vi "DialogAddDesignPattern.vi"(0 "ClassWriterNative":refnum<class "ClassWriterNative.lvclass">, 1 "ClassItemRefIn":refnum<vi>, 5 "error in (no error)":errorcluster) -> (14 "ClassWriterNative":refnum<class "ClassWriterNative.lvclass">, 15 "ClassItemRefOut":refnum<vi>, 16 "AddDesignPatternData":T2, 17 "Cancelled":bool, 19 "error out":errorcluster)   [LabVIEW 2014, in "ClassWriterNative.lvclass"]
uses:
  <resource>/Framework/Providers/Open_GDS/ClassProviders/Provider_LvNativeClass/ClassWriterNative_class/ClassWriterNative.lvclass
  <resource>/Framework/Providers/Open_GDS/ClassProviders/Provider_BaseClassInterface/AddDesignPatternData.ctl
  <resource>/Framework/Providers/Open_GDS/SubVIs/GOOP_HelpButton.ctl
  <resource>/Framework/Providers/Open_GDS/ClassProviders/Provider_BaseClassInterface/DesignPatternsData.ctl
  <resource>/Framework/Providers/Open_GDS/ClassProviders/Common/LvClass_class/GDSLvClass_PlugIn.ctl
  <resource>/Framework/Providers/Open_GDS/ClassProviders/Common/LvClass_class/GDSLvClass_PlugInTypes.ctl
  <resource>/Framework/Providers/Open_GDS/ClassProviders/Provider_BaseClassInterface/BaseProvider_SubVIs/BaseProvider_DesignPatternsActions.ctl
panel:
  out "ProductPicture":picture
  out "TextError":string
  out "_Description":string caption="Description"
  in  "_DesignPatterns":string(tree) caption="Design Patterns"
  out "_ClassTemplateUsed":string caption="Class Template Used"
  out "_ClassProviderName":string caption="Class Provider Name"
  out "_ClassName":string caption="Class name"
  in  "_HelpCreateMethod":T1
  in  "_Help":bool
  in  "_Cancel":bool
  in  "_Next>>":bool
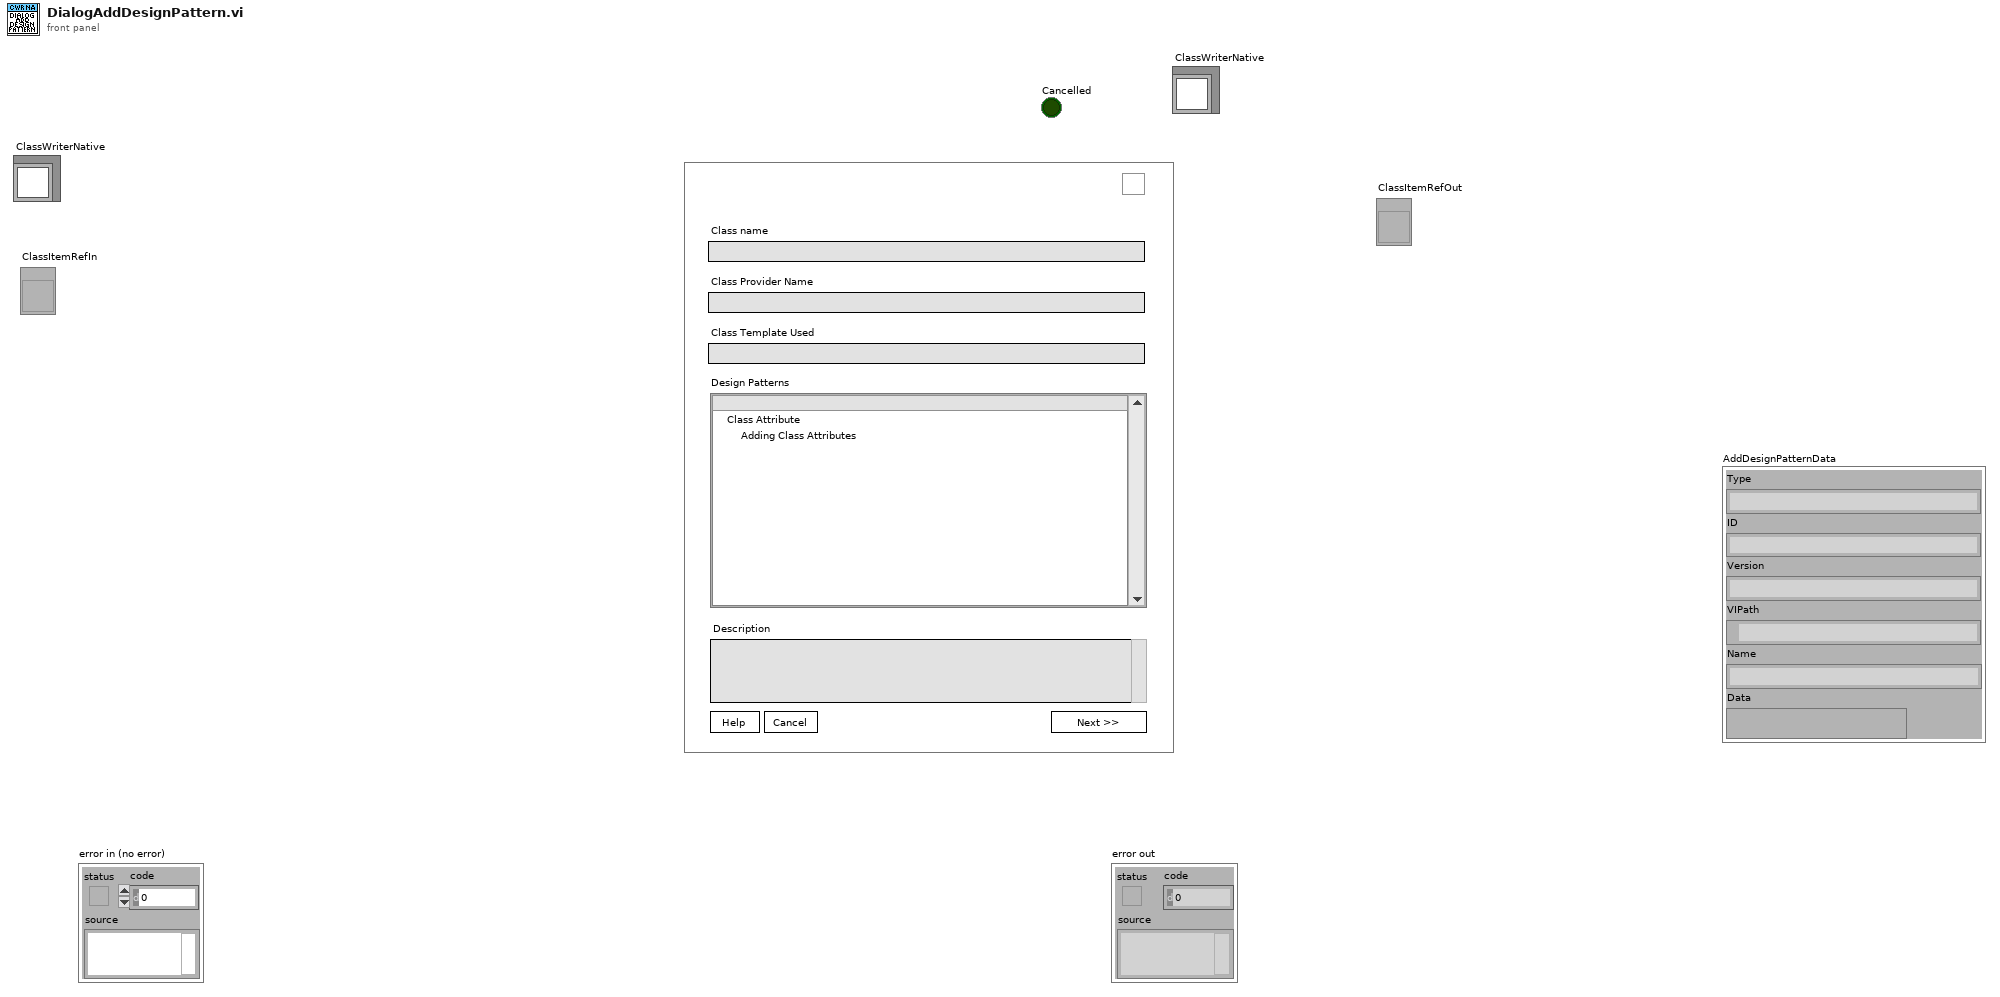
[diagram p1: front panel]
types:
  T1 = typedef "GOOP_HelpButton.ctl" = bool
  T2 = typedef "AddDesignPatternData.ctl" = cluster{"Type":string, "ID":string, "Version":string, "VIPath":path, "Name":string, "Data":variant}
  T3 = typedef "DesignPatternsData.ctl" = cluster{"Type":string, "Patterns":cluster{"ID":string, "Path":path, "Name":string, "Desc":string, "Version":string, "DependenciesID":string[], "OnlyOne":bool}[]}
  T4 = cluster{"Cancel":bool, "ClassProviderName":string, "ClassTemplateUsed":string, "DesignPatterns":T3[], "DataOut":variant, "PlugInVI":path, "DesignPatternID":string, "DesignPatternType":string, "PlugInIDs":string[], "DesignPatternVer":string, "Name":string}
  T5 = typedef "BaseProvider_DesignPatternsActions.ctl" = enum16{"AddPatternDialog", "GeneratePattern", "RemovePattern", "CreatePatternMethod", "UpdatePattern"}
  T6 = typedef "GDSLvClass_PlugIn.ctl" = cluster{"Type":T7, "ID":string, "Version":string, "Path":path, "Name":string, "Data":variant}
  T7 = typedef "GDSLvClass_PlugInTypes.ctl" = enum16{"DesignPattern", "MethodTypes"}
  T8 = typedef "GDSLvCLass_ClassSettingsType.ctl" = cluster{"ClassProviderName":string, "ClassTemplateUsed":string, "ClassTemplateVersion":string, "ClassDescription":string, "PlugIns":T6[], "ConnectorPanePattern":string}
  T9 = cluster{"ID":string, "Path":path, "Name":string, "Desc":string, "Version":string, "DependenciesID":string[], "OnlyOne":bool}[]
  T10 = cluster{"ID":string, "Path":path, "Name":string, "Desc":string, "Version":string, "DependenciesID":string[], "OnlyOne":bool}
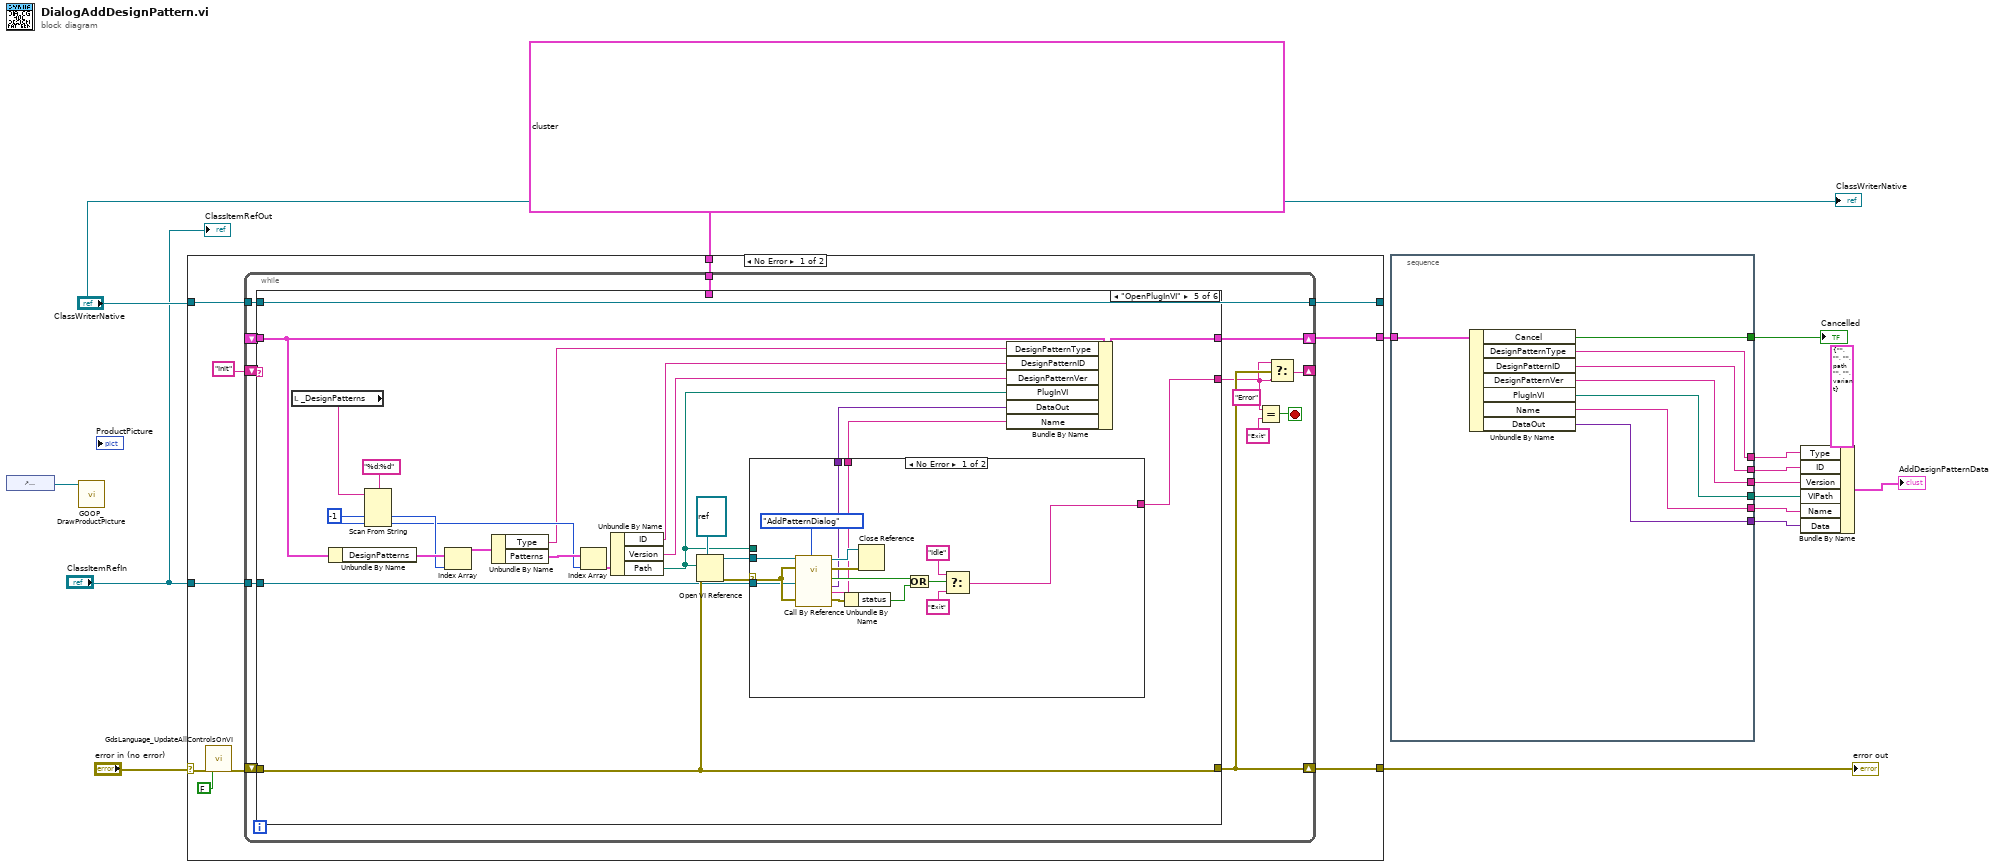
[diagram p0: block diagram]
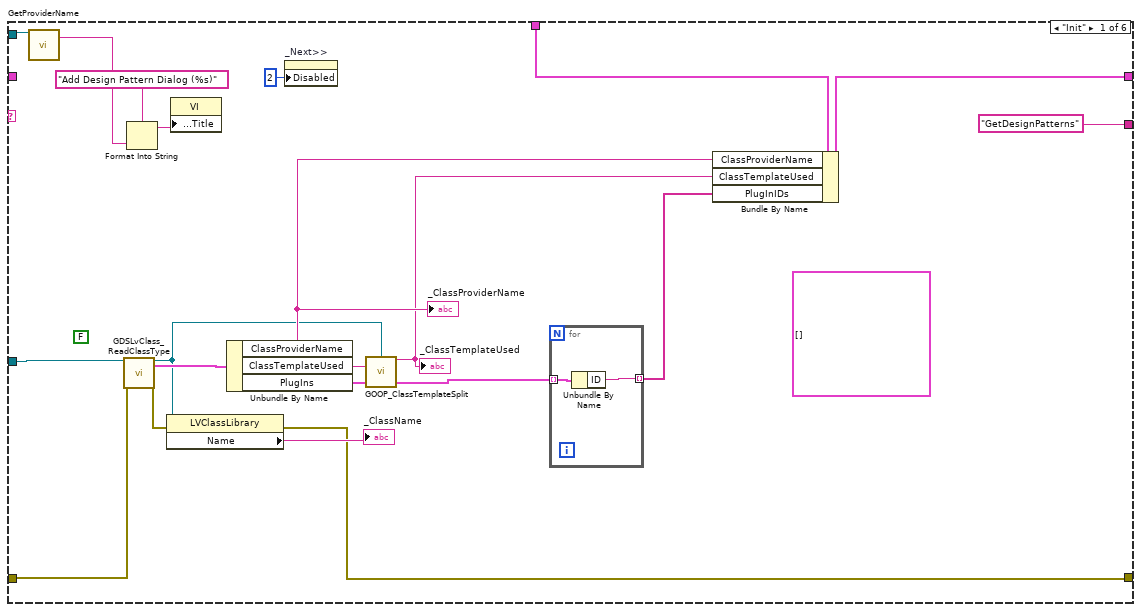
[diagram p2: hidden frame]
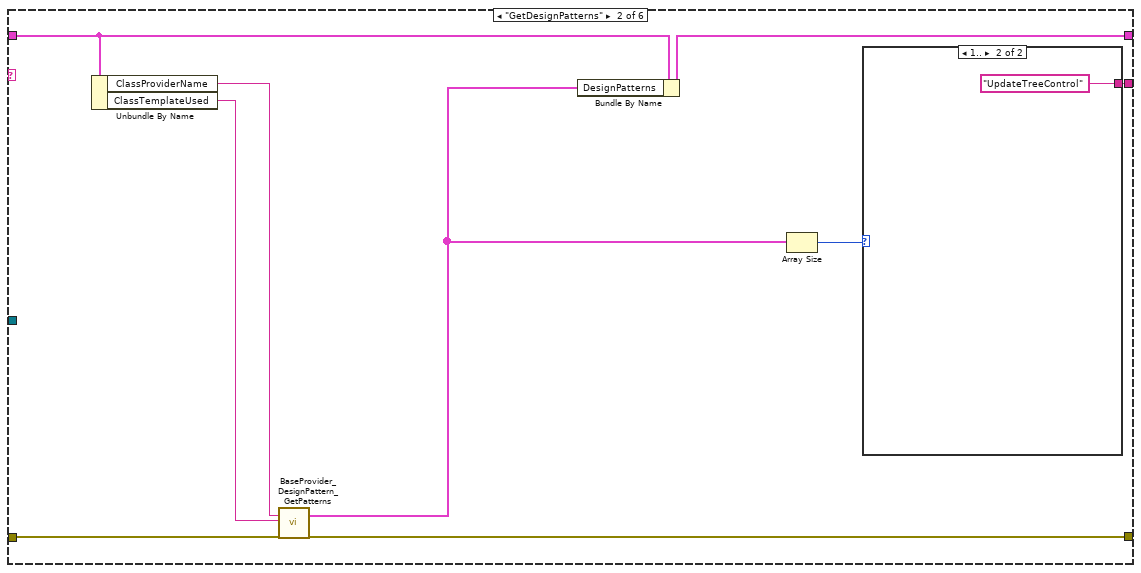
[diagram p3: hidden frame]
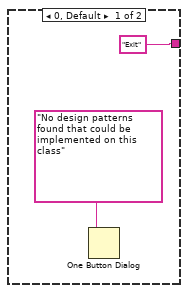
[diagram p4: hidden frame]
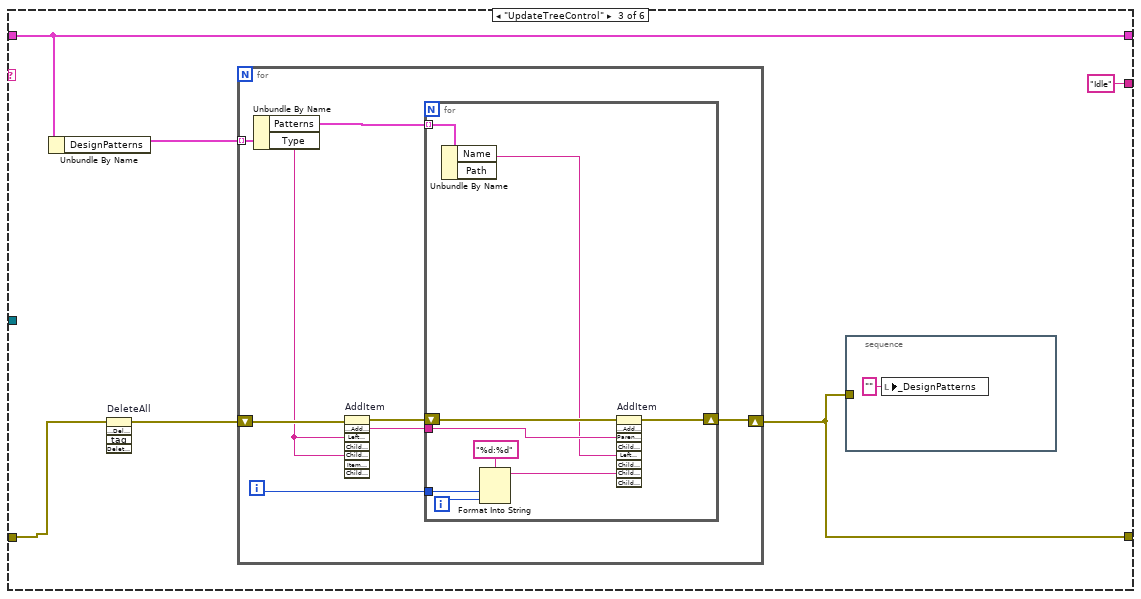
[diagram p5: hidden frame]
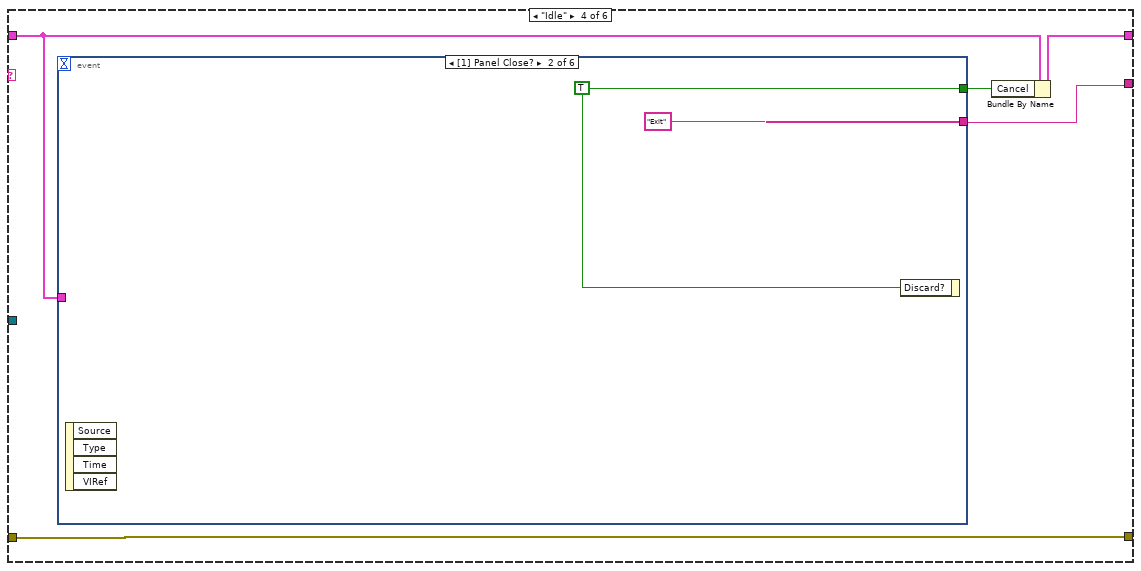
[diagram p6: hidden frame]
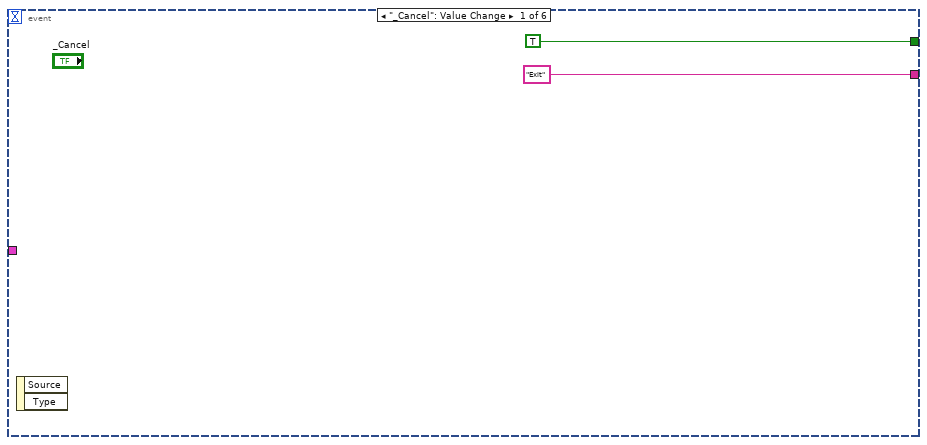
[diagram p7: hidden frame]
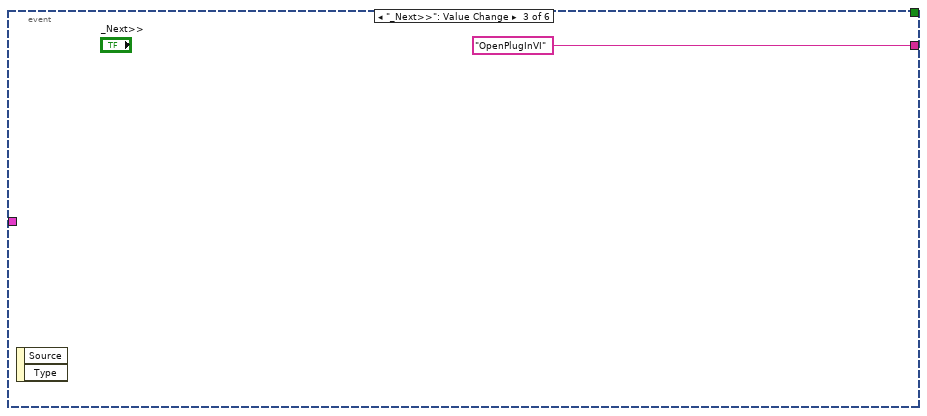
[diagram p8: hidden frame]
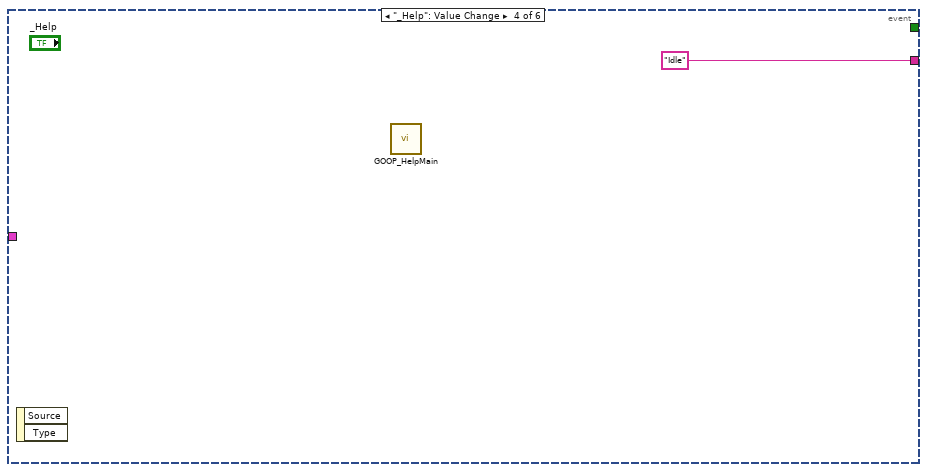
[diagram p9: hidden frame]
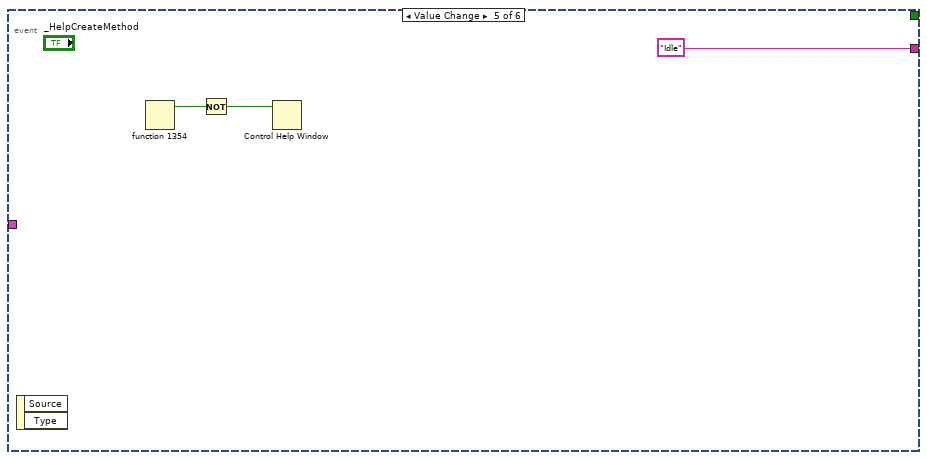
[diagram p10: hidden frame]
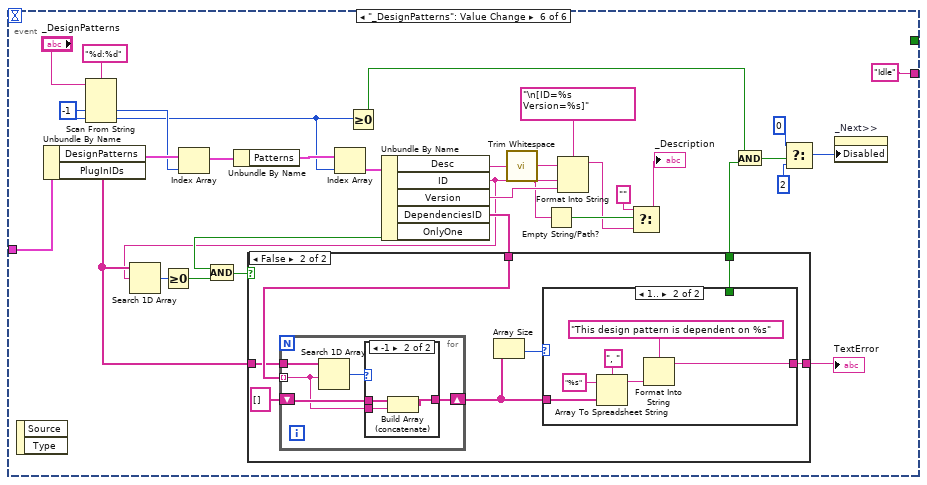
[diagram p11: hidden frame]
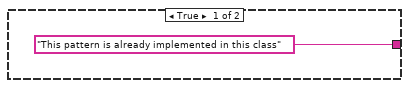
[diagram p12: hidden frame]
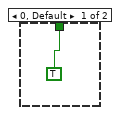
[diagram p13: hidden frame]
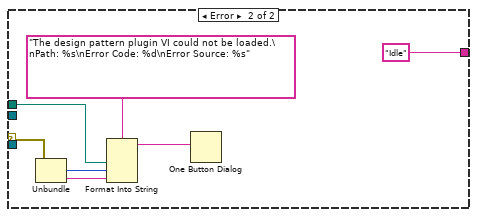
[diagram p15: hidden frame]
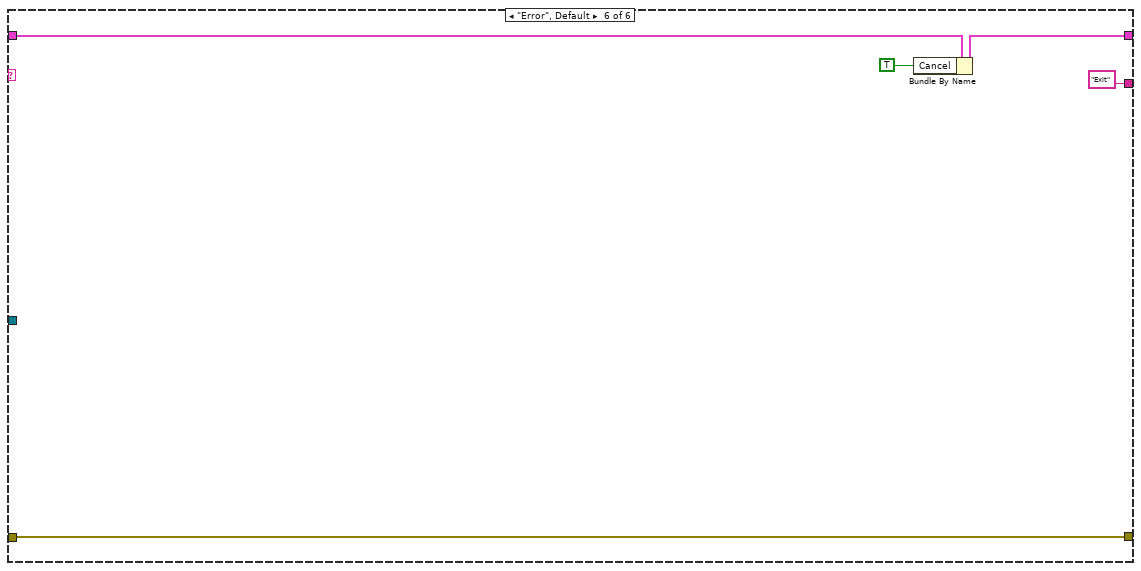
[diagram p16: hidden frame]
diagram:
  n1 = control-ref of="ProductPicture"() -> (w1:refnum<vi>)
  n2 = call <resource>:"GOOP_DrawProductPicture.vi"("ProductPictureControl"=w1) -> ()  [unwired: 10 in, 1 out]
  n3 = case shown="No Error" "error in (no error)" {
    selector: "error in (no error)" -> [w19 w220]
    tunnel: "ClassWriterNative" -> [w23 w219]
    tunnel: [w26 w220] -> w13
    tunnel: [w24 w219] -> _
    tunnel: T4 {"Cancel"=FALSE, "ClassProviderName"="", "ClassTemplateUsed"="", "DesignPatterns"=[], "DataOut"=variant, "PlugInVI"=path "", "DesignPatternID"="", "DesignPatternType"="", "PlugInIDs"=[], "DesignPatternVer"="", "Name"=""} ("output cluster") -> [w22 _]
    tunnel: "ClassItemRefIn" -> [w21 _]
    tunnel: [w20 _] -> w15
    frame No Error {
      n4 = call <resource>:"GdsLanguage_UpdateAllControlsOnVI.vi"("error in (no error)"=w19, "CreateLanguageFile(Use this to create a languageFile)"=FALSE) -> ("error out"=w18:errorcluster)  [unwired: 16 in, 1 out]
      n5 = while {
        shift-right: [w33] -> w26
        shift-left: w18 -> [w39]
        shift-right: [w32] -> _
        shift-left: "Init" -> [w36]
        shift-right: [w37] -> w20
        shift-left: _ -> [w38]
        tunnel: w23 -> [w29]
        tunnel: [w29] -> w24
        tunnel: w22 -> [w28]
        tunnel: w21 -> [w27]
        stop <- w34 stop-if-true
        n6 = case shown="\"OpenPlugInVI\"" w36 {
          tunnel: w38 -> [_ w63 w78 w98 w181 w216]
          tunnel: [w45 w62 w78 w100 w179 w215] -> w37
          tunnel: w39 -> [w52 w68 w77 w102 w178 w217]
          tunnel: [w48 w65 w74 w102 w178 w217] -> w33
          tunnel: w29 -> [w55 _ _ _ _ _]
          tunnel: ["GetDesignPatterns" w70 "Idle" w101 w176 "Exit"] -> w31
          tunnel: w28 -> [w46 _ _ _ _ _]
          tunnel: w27 -> [w53 _ _ _ w173 _]
          frame "Init" {
            (unwired) T6[] [] ("PlugIns")
            (unwired) FALSE ("Visible")
            n7 = call-dynamic "GetProviderName.vi"("ClassWriterNative in"=w55) -> ("ProviderName"=w54:string)  [unwired: 16 in, 2 out]
            n8 = call <resource>:"GDSLvClass_ReadClassType.vi"("Class Refnum In"=w53, "error in (no error)"=w52) -> ("Class Refnum Out"=w40:refnum<vi>, "ClassSettings"=w51:T8, "error out"=w49:errorcluster)  [unwired: 15 in]
            n9 = Format Into String(format string="Add Design Pattern Dialog (%s)", w54) -> (resulting string=w57:string)  [unwired: 2 in, 1 out]
            n10 = property class="LVClassLibrary"(reference=w40, error in=w49) -> (error out=w48:errorcluster, "Name"=→"_ClassName":string)  [unwired: 1 out]
            n11 = property class="VI"("Front Panel.Title"=w57) -> ()  [unwired: 2 in, 2 out]
            n12 = Unbundle By Name(w51) -> ("ClassProviderName"=w47:string, "ClassTemplateUsed"=w42:string, "PlugIns"=w44:T6[])
            "_ClassProviderName" <- w47
            n13 = property on="_Next>>" class="Bool"("Disabled"=u8 2) -> ()  [unwired: 2 in, 2 out]
            n14 = call <resource>:"GOOP_ClassTemplateSplit.vi"("ClassItemRefIn"=w40, "FullClassTemplate"=w42) -> ("StandardTemplate"=w41:string)  [unwired: 12 in, 1 out]
            "_ClassTemplateUsed" <- w41
            n15 = for {
              tunnel: w44 -> [w61] mode=indexing
              tunnel: [w60] -> w43 mode=indexing
              n16 = Unbundle By Name(w61) -> ("ID"=w60:string)
            }
            n17 = Bundle By Name(cluster=w46, "ClassProviderName"=w47, "ClassTemplateUsed"=w41, "PlugInIDs"=w43) -> (w45:T4)
          }
          frame "GetDesignPatterns" {
            n18 = Unbundle By Name(w63) -> ("ClassProviderName"=w67:string, "ClassTemplateUsed"=w66:string)
            n19 = call <resource>:"BaseProvider_DesignPattern_GetPatterns.vi"("FilterOnProviders(Ignored If Empty)"=w67, "FilterOnTemplate(Ignored If Empty)"=w66, "error in (no error)"=w68) -> ("DesignPatterns"=w64:T3[], "error out"=w65:errorcluster)  [unwired: 15 in]
            n20 = Bundle By Name(cluster=w63, "DesignPatterns"=w64) -> (w62:T4)
            n21 = Array Size(array=w64) -> (size(s)=w69:i32)
            n22 = case shown="1.." w69 {
              tunnel: ["Exit" "UpdateTreeControl"] -> w70
              frame 0, Default {
                n23 = One Button Dialog(message="No design patterns found that could be implemented on this class" ("format string")) -> ()  [unwired: 1 in, 1 out]
              }
              frame 1.. {
              }
            }
          }
          frame "UpdateTreeControl" {
            n24 = Unbundle By Name(w78) -> ("DesignPatterns"=w75:T3[])
            n25 = invoke on="DeleteAll" class="Tree (strict)" method="Edit Tree Items.Delete"(error in=w77) -> (error out=w76:errorcluster)  [unwired: 4 in, 4 out]
            n26 = for {
              shift-right: [w81] -> w74
              shift-left: w76 -> [w88]
              tunnel: w75 -> [w87] mode=indexing
              i -> [w82]
              n27 = Unbundle By Name(w87) -> ("Patterns"=w83:T9, "Type"=w84:string)
              n28 = invoke on="AddItem" class="Tree (strict)" method="Edit Tree Items.Add Item to End"(error in=w88, "Left Cell"=w84, "Child Tag"=w84) -> (error out=w86:errorcluster, "Edit Tree Items:Add Item to End"=w85:string)  [unwired: 5 in, 6 out]
              n29 = for {
                shift-right: [w89] -> w81
                shift-left: w86 -> [w96]
                tunnel: w85 -> [w97]
                tunnel: w83 -> [w95] mode=indexing
                tunnel: w82 -> [w92]
                i -> [w91]
                n30 = Unbundle By Name(w95) -> ("Name"=w94:string)  [unwired: 1 out]
                n31 = Format Into String(format string="%d:%d", w92, w91) -> (resulting string=w90:string)  [unwired: 2 in, 1 out]
                n32 = invoke on="AddItem" class="Tree (strict)" method="Edit Tree Items.Add Item"(error in=w96, "Parent Tag"=w97, "Left Cell"=w94, "Child Tag"=w90) -> (error out=w89:errorcluster)  [unwired: 5 in, 8 out]
              }
            }
            n33 = stacked-sequence {
              tunnel: w74 -> [_]
              frame #0 {
                n34 = local write "_DesignPatterns"("" ("_DesignPatterns")) -> ()
              }
            }
          }
          frame "Idle" {
            n35 = event shown="[1] Panel Close?" {
              selector: _ -> [_ _ _ _ _ _]
              dyn-events: _ -> [_ _ _ _ _ _]
              timeout: _ -> [_ _ _ _ _ _]
              tunnel: ["Exit" "Exit" "OpenPlugInVI" "Idle" "Idle" "Idle"] -> w101
              tunnel: [TRUE w105 _ _ _ _] -> w99
              tunnel: w98 -> [_ _ _ _ _ w143]
              event "_Cancel": Value Change {
                n36 = event-data() -> ()  [unwired: 1 in, 2 out]
              }
              event Panel Close? {
                w105 = TRUE
                n37 = event-data() -> ()  [unwired: 1 in, 4 out]
                n38 = event-data("Discard?"=w105) -> ()  [unwired: 1 in, 1 out]
              }
              event "_Next>>": Value Change {
                n39 = event-data() -> ()  [unwired: 1 in, 2 out]
              }
              event "_Help": Value Change {
                n40 = event-data() -> ()  [unwired: 1 in, 2 out]
                n41 = call <resource>:"GOOP_HelpMain.vi"() -> ()  [unwired: 12 in]
              }
              event Value Change {
                n42 = event-data() -> ()  [unwired: 1 in, 2 out]
                n43 = fn#1354() -> (1:w111:bool)  [unwired: 1 out]
                n44 = Not(x=w111) -> (.not. x?=w110:bool)
                n45 = Control Help Window(1:w110) -> ()  [unwired: 1 in]
              }
              event "_DesignPatterns": Value Change {
                w131 = -1 ("default value 1")
                n46 = event-data() -> ()  [unwired: 1 in, 2 out]
                n47 = Unbundle By Name(w143) -> ("DesignPatterns"=w142:T3[], "PlugInIDs"=w121:string[])
                n48 = Scan From String(format string="%d:%d", input string="_DesignPatterns", default 1=w131, default 2=w131) -> (output 1=w141:i32, output 2=w138:i32)  [unwired: 2 in, 3 out]
                n49 = Index Array(array=w142, index=w141) -> (element=w140:T3)
                n50 = Unbundle By Name(w140) -> ("Patterns"=w139:T9)
                n51 = Index Array(array=w139, index=w138) -> (element=w136:T10)
                n52 = Greater Or Equal To 0?(x=w138) -> (x >= 0?=w126:bool)
                n53 = Unbundle By Name(w136) -> ("Desc"=w130:string, "ID"=w115:string, "Version"=w123:string, "DependenciesID"=w128:string[], "OnlyOne"=w117:bool)
                n54 = Search 1D Array(1D array=w121, element=w115) -> (index of element=w120:i32)  [unwired: 1 in]
                n55 = Greater Or Equal To 0?(x=w120) -> (x >= 0?=w119:bool)
                n56 = Compound Arithmetic op=AND(w117, w119) -> (w118:bool)
                n57 = case shown="False" w118 {
                  tunnel: w128 -> [_ w152]
                  tunnel: ["This pattern is already implemented in this class" w149] -> w127
                  tunnel: [_ w147] -> w124
                  tunnel: w121 -> [_ w146]
                  frame True {
                  }
                  frame False {
                    n58 = for {
                      tunnel: w152 -> [w161] mode=indexing
                      tunnel: w146 -> [w164]
                      shift-right: [w160] -> w150
                      shift-left: string[] [] -> [w162]
                      n59 = Search 1D Array(1D array=w164, element=w161) -> (index of element=w163:i32)  [unwired: 1 in]
                      n60 = case shown="-1" w163 {
                        tunnel: w162 -> [w165 w168]
                        tunnel: w161 -> [_ w167]
                        tunnel: [w165 w166] -> w160
                        frame Default {
                        }
                        frame -1 {
                          n61 = Build Array (concatenate)(w168, w167) -> (w166:string[])
                        }
                      }
                    }
                    n62 = Array Size(array=w150) -> (size(s)=w148:i32)
                    n63 = case shown="1.." w148 {
                      tunnel: w150 -> [_ w159]
                      tunnel: [_ w154] -> w149
                      tunnel: [TRUE _] -> w147
                      frame 0, Default {
                      }
                      frame 1.. {
                        n64 = Array To Spreadsheet String(delimiter (Tab)=", ", array=w159, 3:"%s" ("format string")) -> (spreadsheet string=w156:string)
                        n65 = Format Into String(format string="This design pattern is dependent on %s", w156) -> (resulting string=w154:string)  [unwired: 2 in, 1 out]
                      }
                    }
                  }
                }
                "TextError" <- w127
                n66 = call <vilib>:"Trim Whitespace.vi"("string"=w130) -> ("trimmed string"=w129:string)  [unwired: 1 in]
                n67 = Empty String/Path?(string/path=w115) -> (empty?=w116:bool)
                n68 = Format Into String(format string="\n[ID=%s Version=%s]", initial string=w129, w115, w123) -> (resulting string=w114:string)  [unwired: 1 in, 1 out]
                n69 = Select(t="" ("ID"), s=w116, f=w114) -> (s? t:f=→"_Description":string)
                n70 = And(x=w126, y=w124) -> (x .and. y?=w125:bool)
                n71 = Select(t=u8 0, s=w125, f=u8 2 ("Disabled")) -> (s? t:f=w133:u8)
                n72 = property on="_Next>>" class="Bool"("Disabled"=w133) -> ()  [unwired: 2 in, 2 out]
              }
            }
            n73 = Bundle By Name(cluster=w98, "Cancel"=w99) -> (w100:T4)
          }
          frame "OpenPlugInVI" {
            w174 = -1 ("default value 1")
            n74 = local read "_DesignPatterns"() -> (w184:string)
            n75 = Unbundle By Name(w181) -> ("DesignPatterns"=w190:T3[])
            n76 = Scan From String(format string="%d:%d", input string=w184, default 1=w174, default 2=w174) -> (output 1=w189:i32, output 2=w186:i32)  [unwired: 2 in, 3 out]
            n77 = Index Array(array=w190, index=w189) -> (element=w188:T3)
            n78 = Unbundle By Name(w188) -> ("Type"=w172:string, "Patterns"=w187:T9)
            n79 = Index Array(array=w187, index=w186) -> (element=w185:T10)
            n80 = Unbundle By Name(w185) -> ("ID"=w171:string, "Version"=w170:string, "Path"=w175:path)
            n81 = Open VI Reference(type specifier VI Refnum (for type only)=refnum<vi> refnum, vi path=w175, error in (no error)=w178) -> (vi reference=w182:refnum<vi>, error out=w177:errorcluster)  [unwired: 3 in]
            n82 = case shown="No Error" w177 {
              selector: w177 -> [w198 w211]
              tunnel: w182 -> [w206 _]
              tunnel: [w199 _] -> w180
              tunnel: w175 -> [_ w208]
              tunnel: [w196 "Idle"] -> w176
              tunnel: w173 -> [w194 _]
              tunnel: [w192 _] -> w169
              frame No Error {
                n83 = call-by-ref "?"(reference=w206, error in=w198, "Action"=BaseProvider_DesignPatternsActions."AddPatternDialog", 8:"error in (no error)"=w198, "ClassRefToActOn"=w194) -> (reference out=w201:refnum<vi>, error out=w202:errorcluster, 0:"error out"=w205:errorcluster, "Name"=w192:string, "DataOut"=w199:variant, "Cancelled"=w204:bool)  [unwired: 5 in]
                n84 = Unbundle By Name(w205) -> ("status"=w203:bool)
                n85 = Close Reference(reference=w201, error in (no error)=w202) -> ()  [unwired: 1 out]
                n86 = Or(x=w204, y=w203) -> (x .or. y?=w200:bool)
                n87 = Select(t="Idle", s=w200, f="Exit") -> (s? t:f=w196:string)
              }
              frame Error {
                n88 = Unbundle(w211) -> ("code"=w210:i32, "source"=w209:string)  [unwired: 1 out]
                n89 = Format Into String(format string="The design pattern plugin VI could not be loaded.\nPath: %s\nError Code: %d\nError Source: %s" ("message"), w208, w210, w209) -> (resulting string=w212:string)  [unwired: 2 in, 1 out]
                n90 = One Button Dialog(message=w212) -> ()  [unwired: 1 in, 1 out]
              }
            }
            n91 = Bundle By Name(cluster=w181, "DesignPatternType"=w172, "DesignPatternID"=w171, "DesignPatternVer"=w170, "PlugInVI"=w175, "DataOut"=w180, "Name"=w169) -> (w179:T4)
          }
          frame "Error", Default {
            n92 = Bundle By Name(cluster=w216, "Cancel"=TRUE) -> (w215:T4)
          }
        }
        n93 = Equal?(x=w31, y="Exit") -> (x = y?=w34:bool)
        n94 = Select(t="Error", s=w33, f=w31) -> (s? t:f=w32:string)
      }
    }
    frame Error {
    }
  }
  "error out" <- w13
  n95 = stacked-sequence {
    tunnel: w15 -> [w228]
    tunnel: [w227] -> w14
    tunnel: [w226] -> w6
    tunnel: [w225] -> w7
    tunnel: [w224] -> w5
    tunnel: [w223] -> w4
    tunnel: [w222] -> w3
    tunnel: [w221] -> w2
    frame #0 {
      n96 = Unbundle By Name(w228) -> ("Cancel"=w227:bool, "DesignPatternType"=w223:string, "DesignPatternID"=w224:string, "DesignPatternVer"=w222:string, "PlugInVI"=w226:path, "Name"=w221:string, "DataOut"=w225:variant)
    }
  }
  "Cancelled" <- w14
  n97 = Bundle By Name(cluster=T2 {"Type"="", "ID"="", "Version"="", "VIPath"=path "", "Name"="", "Data"=variant} ("AddDesignPatternData"), "Type"=w4, "ID"=w5, "Version"=w3, "VIPath"=w6, "Name"=w2, "Data"=w7) -> (→"AddDesignPatternData":T2)
  "ClassWriterNative" <- "ClassWriterNative"
  "ClassItemRefOut" <- "ClassItemRefIn"
